vi "AMZ_S3_APIHLP_Parse PUT Bucket Request Parameters.vi"(8 "error in (no error)":errorcluster, 11 "PUT Bucket Request parameters":T2) -> (0 "error out":errorcluster, 3 "HTTP Headers":T1[](array[typedef]), 4 "PUT Data":string)   [LabVIEW 2015, in "LV Interface for Amazon S3.lvlib"]
uses:
  LV Interface for Amazon S3.lvlib
  Typedefs/AMZ_S3_API_PUT Bucket Request Parameters.ctl
  Typedefs/AMZ_S3_ACL.ctl
  Typedefs/AMZ_S3_LocationConstraint.ctl
  Typedefs/AMZ_S3_HTTP Header-Value pair.ctl
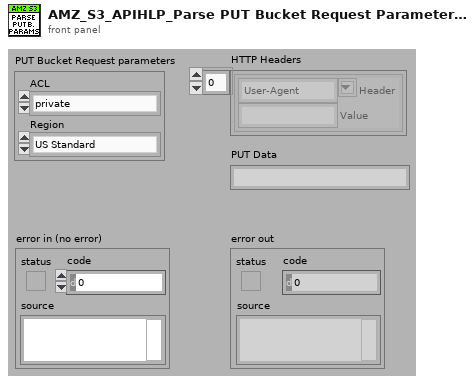
[diagram p1: front panel]
types:
  T1 = typedef "LV Interface for Amazon S3.lvlib/AMZ_S3_HTTP Header-Value pair.ctl" = cluster{"Header":string, "Value":string}
  T2 = typedef "LV Interface for Amazon S3.lvlib/AMZ_S3_API_PUT Bucket Request Parameters.ctl" = cluster{"ACL":T3, "Region":T4}
  T3 = typedef "LV Interface for Amazon S3.lvlib/AMZ_S3_ACL.ctl" = enum16{"private", "public-read", "public-read-write", "aws-exec-read", "authenticated-read", "bucket-owner-read", "bucket-owner-full-control"}
  T4 = typedef "LV Interface for Amazon S3.lvlib/AMZ_S3_LocationConstraint.ctl" = enum16{"US Standard", "us-east-2", "us-west-1", "us-west-2", "ap-northeast-1", "ap-northeast-2", "ap-southeast-1", "ap-southeast-2", "ca-central-1", "eu-central-1", "eu-west-1", "eu-west-2", "sa-east-1"}
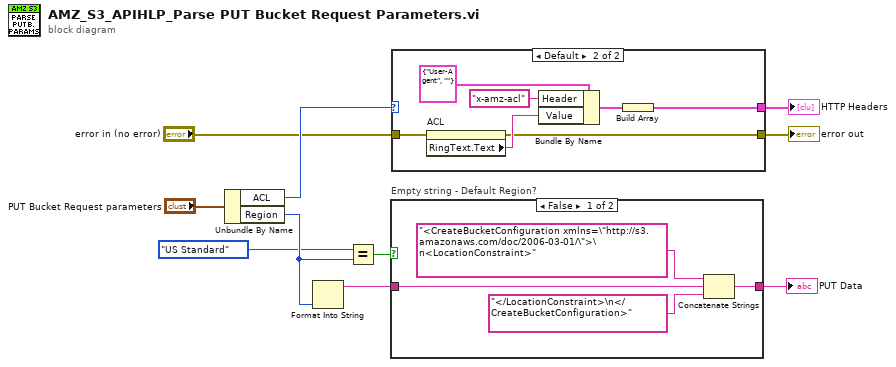
[diagram p0: block diagram]
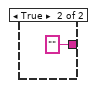
[diagram p2: hidden frame]
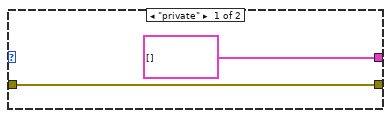
[diagram p3: hidden frame]
diagram:
  n1 = Unbundle By Name("PUT Bucket Request parameters") -> ("ACL"=w9:T3, "Region"=w2:T4)
  n2 = Format Into String(w2) -> (resulting string=w4:string)  [unwired: 3 in, 1 out]
  n3 = Equal?(x=AMZ_S3_LocationConstraint."US Standard", y=w2) -> (x = y?=w3:bool)
  n4 = case "Empty string - Default Region?" shown="False" w3 {
    tunnel: w4 -> [w14 _]
    tunnel: [w11 ""] -> w5
    frame False {
      n5 = Concatenate Strings("<CreateBucketConfiguration xmlns=\"http://s3.amazonaws.com/doc/2006-03-01/\">\n<LocationConstraint>", w14, "</LocationConstraint>\n</CreateBucketConfiguration>") -> (w11:string)
    }
    frame True {
    }
  }
  "PUT Data" <- w5
  n6 = case shown="Default" w9 {
    tunnel: "error in (no error)" -> [w16 w24]
    tunnel: [w16 w20] -> w7
    tunnel: [T1[] [] w18] -> w8
    frame "private" {
    }
    frame Default {
      n7 = property on="ACL" class="Enum (strict)"(error in=w24) -> (error out=w20:errorcluster, "RingText.Text"=w21:string)  [unwired: 1 in, 1 out]
      n8 = Bundle By Name(cluster=T1 {"Header"="User-Agent", "Value"=""} ("HTTP Header-Value pair"), "Header"="x-amz-acl", "Value"=w21) -> (w19:T1)
      n9 = Build Array(w19) -> (w18:T1[])
    }
  }
  "error out" <- w7
  "HTTP Headers" <- w8
